vi "Password_Checker.vi"(8 "error in (no error)":errorcluster, 11 "Password":string) -> (0 "error out":errorcluster, 2 "Password Exist?":bool, 3 "User_ID":i32, 5 "Data":string[][](array[string]))   [LabVIEW 2025]
uses:
  <vilib>/Utility/file.llb/Read Delimited Spreadsheet (string).vi
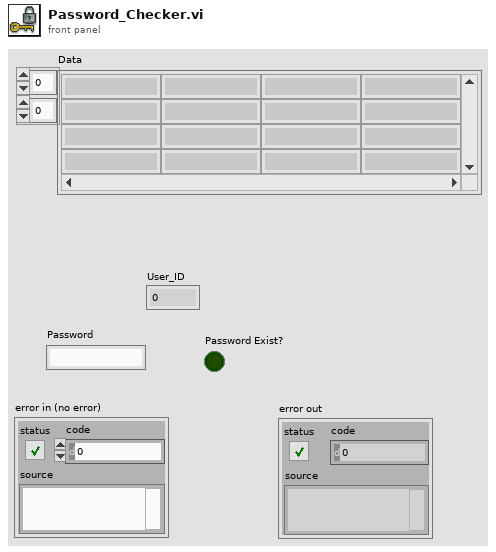
[diagram p1: front panel]
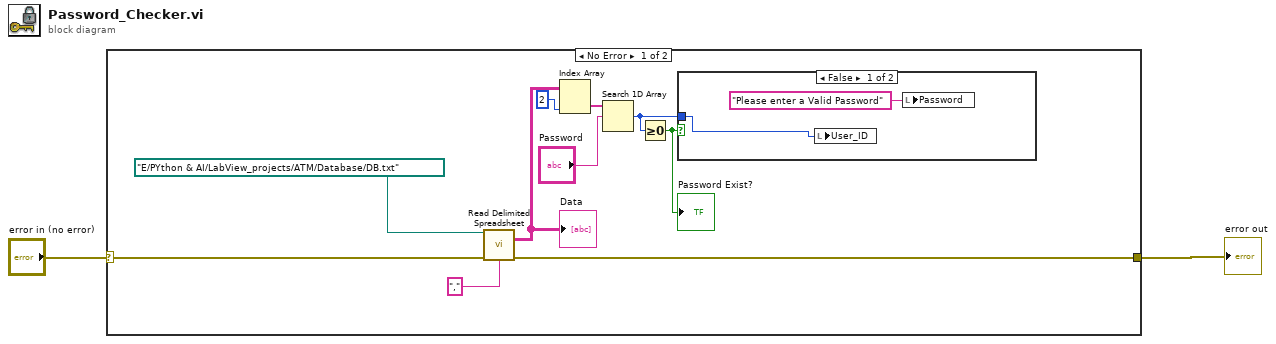
[diagram p0: block diagram]
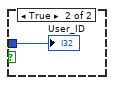
[diagram p2: hidden frame]
diagram:
  n1 = case shown="No Error" "error in (no error)" {
    selector: "error in (no error)" -> [w4 w16]
    tunnel: [w3 w16] -> w1
    frame No Error {
      n2 = call-poly <vilib>:"Read Delimited Spreadsheet.vi"("file path (dialog if empty)"=path "E:/PYthon & AI/LabView_projects/ATM/Database/DB.txt", "error in (no error)"=w4, "delimiter (\\t)"="," ("delimiter (\\t)")) -> ("all rows"=w9:string[][], "error out"=w3:errorcluster)  [unwired: 7 in, 4 out]
      "Data" <- w9
      n3 = Index Array(array=w9, index (col)=2 ("index (row)")) -> (element=w8:string[])  [unwired: 1 in]
      n4 = Search 1D Array(1D array=w8, element="Password") -> (index of element=w5:i32)  [unwired: 1 in]
      n5 = Greater Or Equal To 0?(x=w5) -> (x >= 0?=w6:bool)
      "Password Exist?" <- w6
      n6 = case shown="False" w6 {
        tunnel: w5 -> [w13 w15]
        frame False {
          n7 = local write "User_ID"(w13) -> ()
          n8 = local write "Password"("Please enter a Valid Password" ("Password")) -> ()
        }
        frame True {
          "User_ID" <- w15
        }
      }
    }
    frame Error {
    }
  }
  "error out" <- w1
